vi "Variant to Display String.vi"(3 "Variant":variant) -> (1 "xml string":string)   [LabVIEW 2019, in "RemoteControl.lvclass"]
uses:
  RemoteControl.lvclass
panel:
  out "offset past match":i32
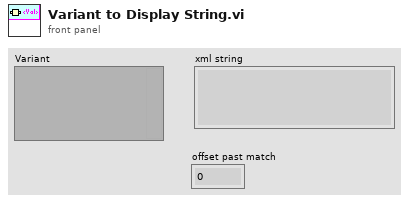
[diagram p1: front panel]
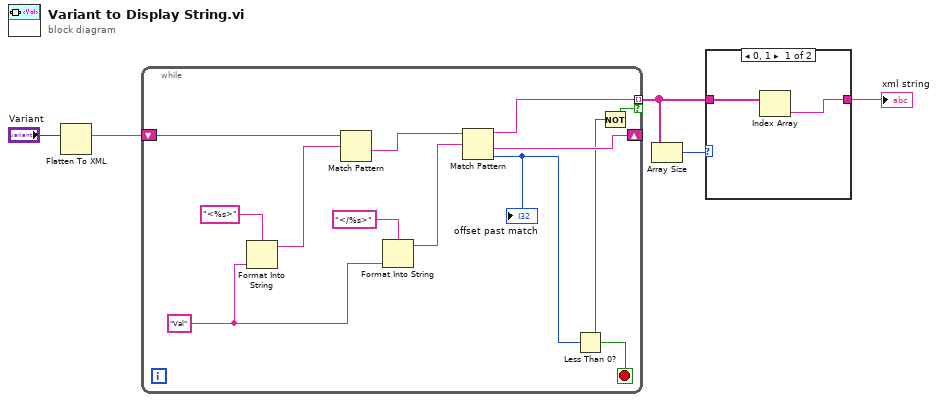
[diagram p0: block diagram]
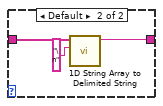
[diagram p2: hidden frame]
diagram:
  n1 = Flatten To XML(anything="Variant") -> (xml string=w5:string)
  n2 = while {
    shift-right: [w10] -> _
    shift-left: w5 -> [w11]
    tunnel: [w9] -> w3 mode=indexing if=w7
    stop <- w6 stop-if-true
    w15 = "Val" ("Tag")
    n3 = Format Into String(format string="<%s>", w15) -> (resulting string=w16:string)  [unwired: 2 in, 1 out]
    n4 = Match Pattern(string=w11, regular expression=w16) -> (after substring=w12:string)  [unwired: 1 in, 3 out]
    n5 = Format Into String(format string="</%s>", w15) -> (resulting string=w17:string)  [unwired: 2 in, 1 out]
    n6 = Match Pattern(string=w12, regular expression=w17) -> (before substring=w9:string, after substring=w10:string, offset past match=w8:i32)  [unwired: 1 in, 1 out]
    "offset past match" <- w8
    n7 = Less Than 0?(x=w8) -> (x < 0?=w6:bool)
    n8 = Not(x=w6) -> (.not. x?=w7:bool)
  }
  n9 = Array Size(array=w3) -> (size(s)=w2:i32)
  n10 = case shown="0, 1" w2 {
    tunnel: [w18 w22] -> w4
    tunnel: w3 -> [w19 w20]
    frame 0, 1 {
      n11 = Index Array(array=w19) -> (element=w18:string)  [unwired: 1 in]
    }
    frame Default {
      n12 = call <vilib>:"1D String Array to Delimited String.vi"("delimiter"="\n", "string array"=w20) -> ("delimited string"=w22:string)  [unwired: 9 in]
    }
  }
  "xml string" <- w4
